vi "build error.vi"(1 "Error code":i32, 2 "Error msg":string, 3 "Trigger error":bool) -> (0 "error out":errorcluster)   [LabVIEW 2018]
panel:
  # "This is a helper vi to build error messages. \nUse it instead of manually sending errors.\n\nThis is a Preallocated Reentrant VI, meaning multiple\nof this VI can be used without a problem with no gitter, \nat the cost of more memory usage."
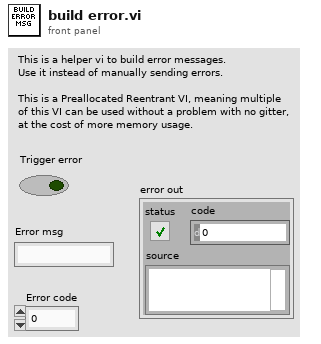
[diagram p1: front panel]
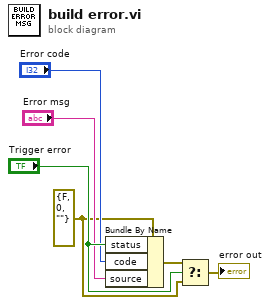
[diagram p0: block diagram]
diagram:
  w3 = errorcluster {"status"=FALSE, "code"=0, "source"=""} ("error constant")
  n1 = Bundle By Name(cluster=w3, "status"="Trigger error", "code"="Error code", "source"="Error msg") -> (w2:errorcluster)
  n2 = Select(t=w2, s="Trigger error", f=w3) -> (s? t:f=→"error out":errorcluster)
